vi "CalibrateStartPosition.vi"(10 "Start Position [mm]":dbl[](array[numeric]), 11 ".NET Refnum In":refnum<k24>) -> (2 "Final Position [mm]":dbl[](array[numeric]))   [LabVIEW 2016]
uses:
  C:/Users/Aerotech/Documents/BNLStaveAssembly-blueprint/Bin/Aerotech.A3200.dll
  BNLStaveAssembly-blueprint/Bin/Aerotech.A3200.dll
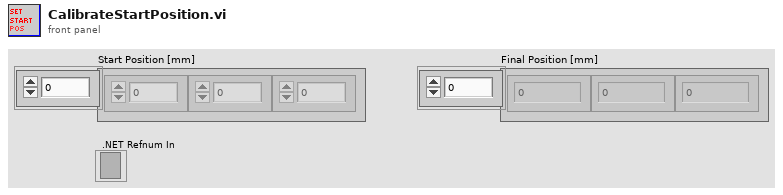
[diagram p1: front panel]
types:
  T1 = cluster{"Final X":dbl, "Final Y":dbl, "Final Z":dbl}
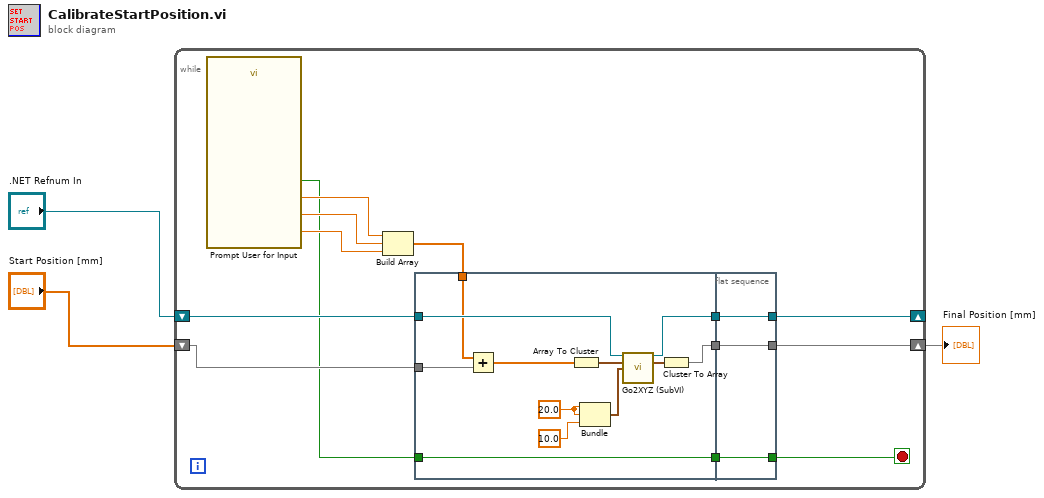
[diagram p0: block diagram]
diagram:
  n1 = while {
    shift-right: [w16] -> w1
    shift-left: "Start Position [mm]" -> [w10]
    shift-right: [w14] -> _
    shift-left: ".NET Refnum In" -> [w15]
    stop <- w4 stop-if-true
    n2 = call "Prompt User for Input"() -> ("Adjust z [mm]"=w11:dbl, "Adjust y [mm]"=w12:dbl, "Adjust x [mm]"=w13:dbl, "Accept"=w8:bool)  [unwired: 14 in, 2 out]
    n3 = Build Array(w13, w12, w11) -> (w9:dbl[])
    n4 = flat-sequence {
      tunnel: w15 -> [w26]
      tunnel: w10 -> [w21]
      tunnel: w9 -> [w20]
      tunnel: w8 -> [w17]
      tunnel: [w27] -> w7
      tunnel: [w25] -> w6
      tunnel: [w17] -> w5
      tunnel: [w29] -> w4
      tunnel: [w30] -> w14
      tunnel: [w31] -> w16
      tunnel: w7 -> [w31]
      tunnel: w6 -> [w30]
      tunnel: w5 -> [w29]
      frame #0 {
        w23 = 20.0
        n5 = Add(x=w20, y=w21) -> (x+y=w22:dbl[])
        n6 = Array To Cluster(array=w22) -> (cluster=w19:cluster{"[0]":dbl, "[1]":dbl, "[2]":dbl})
        n7 = Bundle(w23, w23, 10.0) -> (w24:cluster{dbl, dbl, dbl})  [unwired: 1 in]
        n8 = call "Go2XYZ (SubVI).vi"(".NET Refnum in"=w26, "Go to Coordinates"=w19, "Axis Speeds"=w24) -> (".NET Refnum out"=w25:refnum<k24>, "Final Position"=w28:T1)  [unwired: 8 in, 3 out]
        n9 = Cluster To Array(cluster=w28) -> (array=w27:dbl[])
      }
      frame #1 {
      }
    }
  }
  "Final Position [mm]" <- w1
